vi "Sets and Query the Temperature Unit.vi"(5 "Enable to Query":bool=TRUE, 7 "Enable to Sets":bool=TRUE, 8 "error in":errorcluster, 10 "Temperature Unit":u8(ring) items=["C", "F"], 11 "VISA resource name":refnum<visa-resource-name>) -> (0 "error out":errorcluster, 2 "Return the Temperature Unit":string, 3 "VISA resource name out":refnum<visa-resource-name>)   [LabVIEW 2011, in "DMM4.lvlib"]
uses:
  <instrlib>/DMM4/DMM4.lvlib
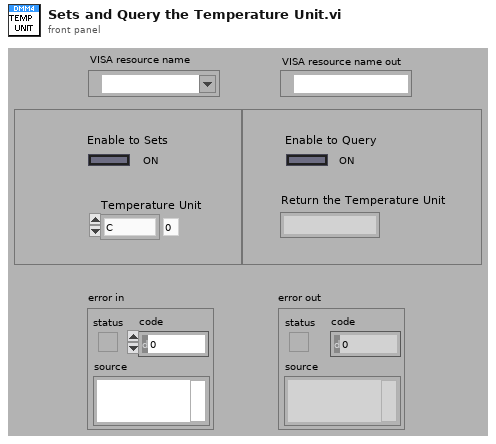
[diagram p1: front panel]
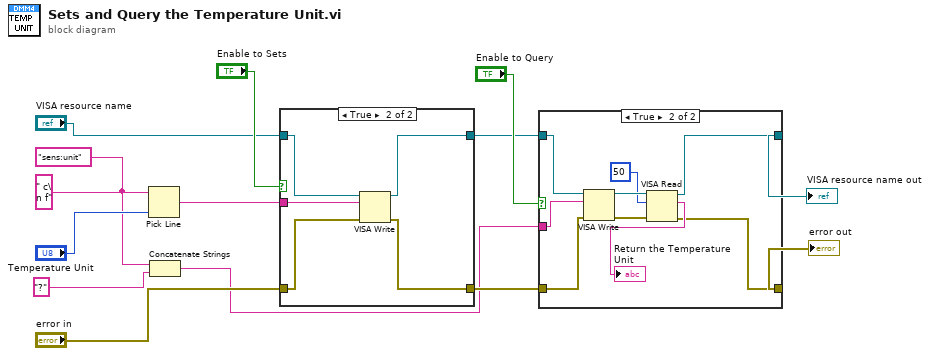
[diagram p0: block diagram]
diagram:
  w10 = "sens:unit"
  n1 = Pick Line(string ("")=w10, multi-line string=" c\n f", line index="Temperature Unit") -> (output string=w9:string)
  n2 = Concatenate Strings(w10, "?") -> (w3:string)
  n3 = case shown="True" "Enable to Sets" {
    tunnel: w9 -> [_ w21]
    tunnel: "VISA resource name" -> [w16 w20]
    tunnel: "error in" -> [w15 w19]
    tunnel: [w16 w18] -> w5
    tunnel: [w15 w17] -> w4
    frame False {
    }
    frame True {
      n4 = VISA Write(VISA resource name=w20, write buffer=w21, error in (no error)=w19) -> (VISA resource name out=w18:refnum<visa-resource-name>, error out=w17:errorcluster)  [unwired: 1 out]
    }
  }
  n5 = case shown="True" "Enable to Query" {
    tunnel: w5 -> [w23 w31]
    tunnel: w4 -> [w22 w30]
    tunnel: w3 -> [_ w32]
    tunnel: [w23 w25] -> w2
    tunnel: [w22 w24] -> w1
    frame False {
    }
    frame True {
      n6 = VISA Write(VISA resource name=w31, write buffer=w32, error in (no error)=w30) -> (VISA resource name out=w29:refnum<visa-resource-name>, error out=w28:errorcluster)  [unwired: 1 out]
      n7 = VISA Read(VISA resource name=w29, byte count=u32 50, error in (no error)=w28) -> (VISA resource name out=w25:refnum<visa-resource-name>, read buffer=→"Return the Temperature Unit":string, error out=w24:errorcluster)  [unwired: 1 out]
    }
  }
  "VISA resource name out" <- w2
  "error out" <- w1
